vi "Execute_Experiment.vi"(2 "Repetition Timing":u32, 3 "Nr of Repetitions":u16, 4 "Start and Stop Index":i16) -> (0 "Error Out":u8, 1 "Aborted":bool)   [LabVIEW 2023]
uses:
  <vilib>/rvi/DataTransferAndStorage/Container/XNode/niFpgaContainer.xnode
  <vilib>/rvi/DataTransferAndStorage/Register/Emulation/niFpgaRegisterEmulation.vi
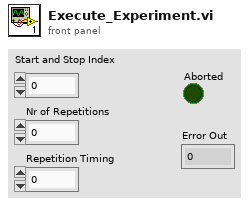
[diagram p1: front panel]
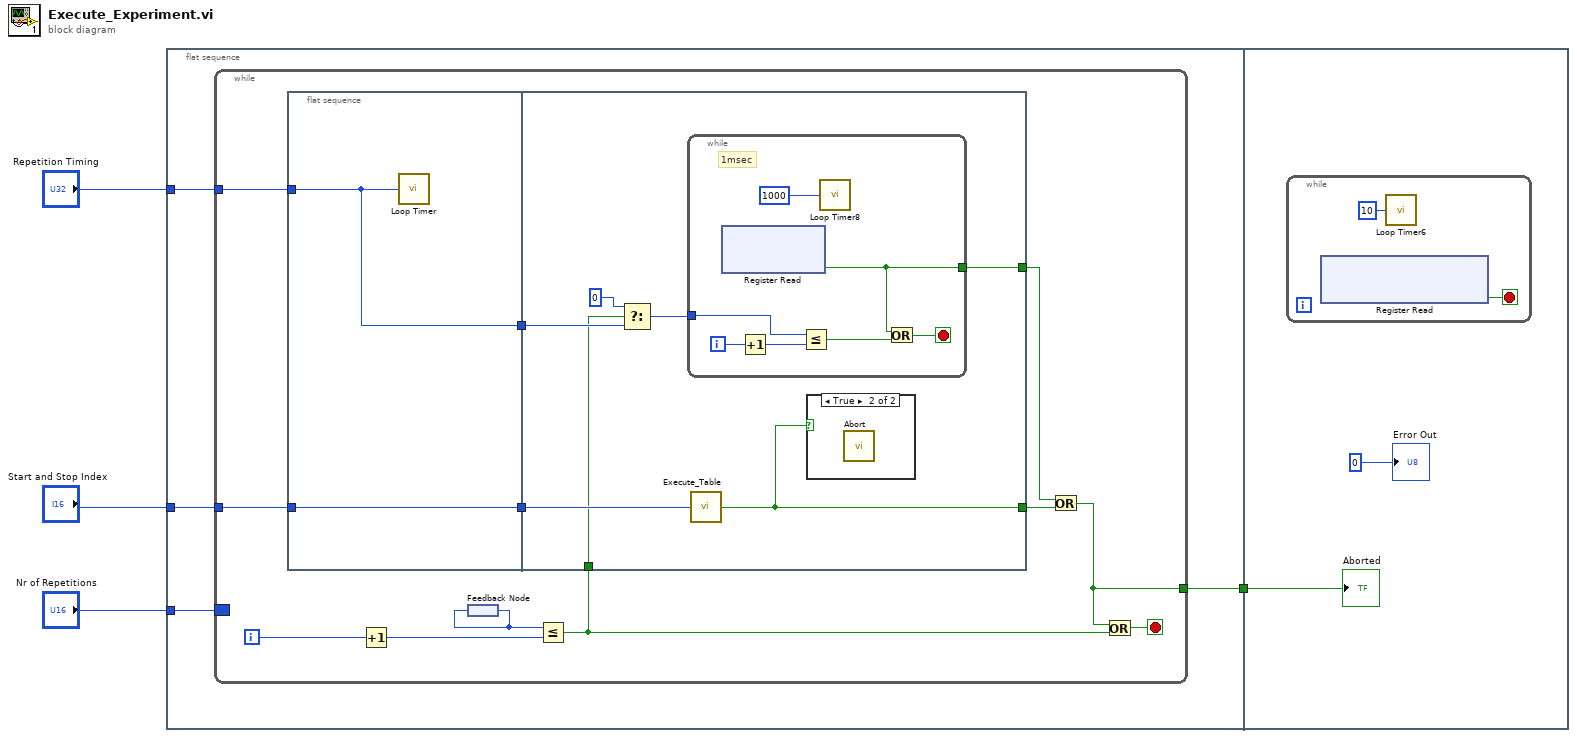
[diagram p0: block diagram]
diagram:
  n1 = flat-sequence {
    tunnel: [w8] -> w4
    tunnel: "Start and Stop Index" -> [w5]
    tunnel: "Repetition Timing" -> [w6]
    tunnel: "Nr of Repetitions" -> [w7]
    tunnel: w4 -> [w38]
    frame #0 {
      n2 = while {
        tunnel: [w10] -> w8
        border: w7 -> [_]
        tunnel: w6 -> [w16]
        tunnel: w5 -> [w14]
        i -> [w19]
        stop <- w20 stop-if-true
        n3 = flat-sequence {
          tunnel: w16 -> [w22]
          tunnel: [w22] -> w15
          tunnel: w14 -> [w21]
          tunnel: [w21] -> w13
          tunnel: w15 -> [w26]
          tunnel: w13 -> [w29]
          tunnel: [w27] -> w12
          tunnel: [w28] -> w11
          tunnel: w9 -> [w25]
          frame #0 {
            n4 = call "Loop Timer"("Count(mSec)"=w22) -> ()  [unwired: 1 out]
          }
          frame #1 {
            n5 = Select(t=u32 0, s=w25, f=w26) -> (s? t:f=w24:u32)
            n6 = while {
              tunnel: w24 -> [w36]
              tunnel: [w32] -> w28
              i -> [w35]
              stop <- w33 stop-if-true
              # "1msec"
              n7 = xnode ("Register Read")() -> ("Data"=w32:bool)  [unwired: 1 in, 1 out]
              n8 = Increment(x=w35) -> (x+1=w30:i32)
              n9 = Less Or Equal?(x=w36, y=w30) -> (x <= y?=w34:bool)
              n10 = call "Loop Timer8"("Count(uSec)"=u32 1000 ("Count(Ticks)")) -> ()  [unwired: 1 out]
              n11 = Or(x=w32, y=w34) -> (x .or. y?=w33:bool)
            }
            n12 = call "Execute_Table.vi"("Start and Stop Indexes"=w29) -> ("Aborted"=w27:bool)
            n13 = case shown="True" w27 {
              frame False {
              }
              frame True {
                n14 = call "Abort.vi"() -> ()  [unwired: 12 in]
              }
            }
          }
        }
        n15 = Increment(x=w19) -> (x+1=w17:i32)
        n16 = feedback #1() -> (w18:u16)
        n17 = feedback-in #1(w18) -> ()
        n18 = Less Or Equal?(x=w18, y=w17) -> (x <= y?=w9:bool)
        n19 = Or(x=w11, y=w12) -> (x .or. y?=w10:bool)
        n20 = Or(x=w10, y=w9) -> (x .or. y?=w20:bool)
      }
    }
    frame #1 {
      n21 = while {
        stop <- w39 stop-if-true
        n22 = xnode ("Register Read")() -> ("Data"=w39:bool)  [unwired: 1 in, 1 out]
        n23 = call "Loop Timer6"("Count(uSec)"=u8 10) -> ()  [unwired: 1 out]
      }
      "Aborted" <- w38
      "Error Out" <- i16 0
    }
  }
